vi "sub_Main Robot.vi"() -> ()   [LabVIEW 2017]
uses:
  <vilib>/Analysis/Matrix/Datatypes/RealMatrix.ctl
  <vilib>/Analysis/baseanly.llb/Mean (DBL).vi
  <vilib>/Analysis/baseanly.llb/A x Vector.vi
  <vilib>/DAQmx/read.llb/DAQmx Read (Analog 2D DBL NChan NSamp).vi
  <vilib>/DAQmx/create/channels.llb/DAQmx Create Channel (AI-Voltage-Basic).vi
  <vilib>/DAQmx/configure/timing.llb/DAQmx Timing (Sample Clock).vi
  <vilib>/DAQmx/miscellaneous.llb/DAQmx Fill In Error Info.vi
  <vilib>/Analysis/3filter.llb/Butterworth Filter (DBL).vi
  <vilib>/Analysis/NI_AALBase.lvlib
  <vilib>/Analysis/Matrix/NI_Matrix.lvlib
panel:
  in  "Calibration Matrix":T1
  out "Waveform Chart":T2(graph)
  out "Waveform Graph":dbl[][](graph)
  in  "stop":bool
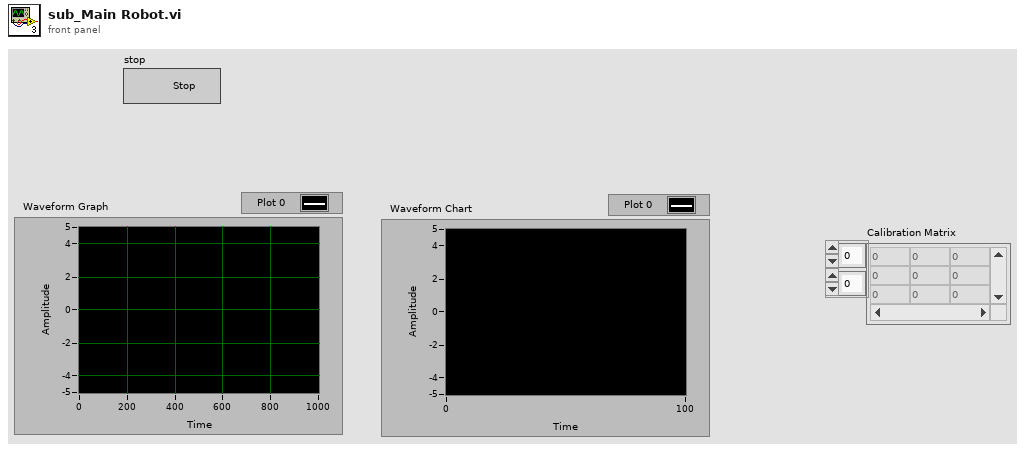
[diagram p1: front panel]
types:
  T1 = typedef "NI_Matrix.lvlib/RealMatrix.ctl" = dbl[][]
  T2 = cluster{"mean":dbl, "mean":dbl, "mean":dbl, "mean":dbl, "mean":dbl, "mean":dbl}
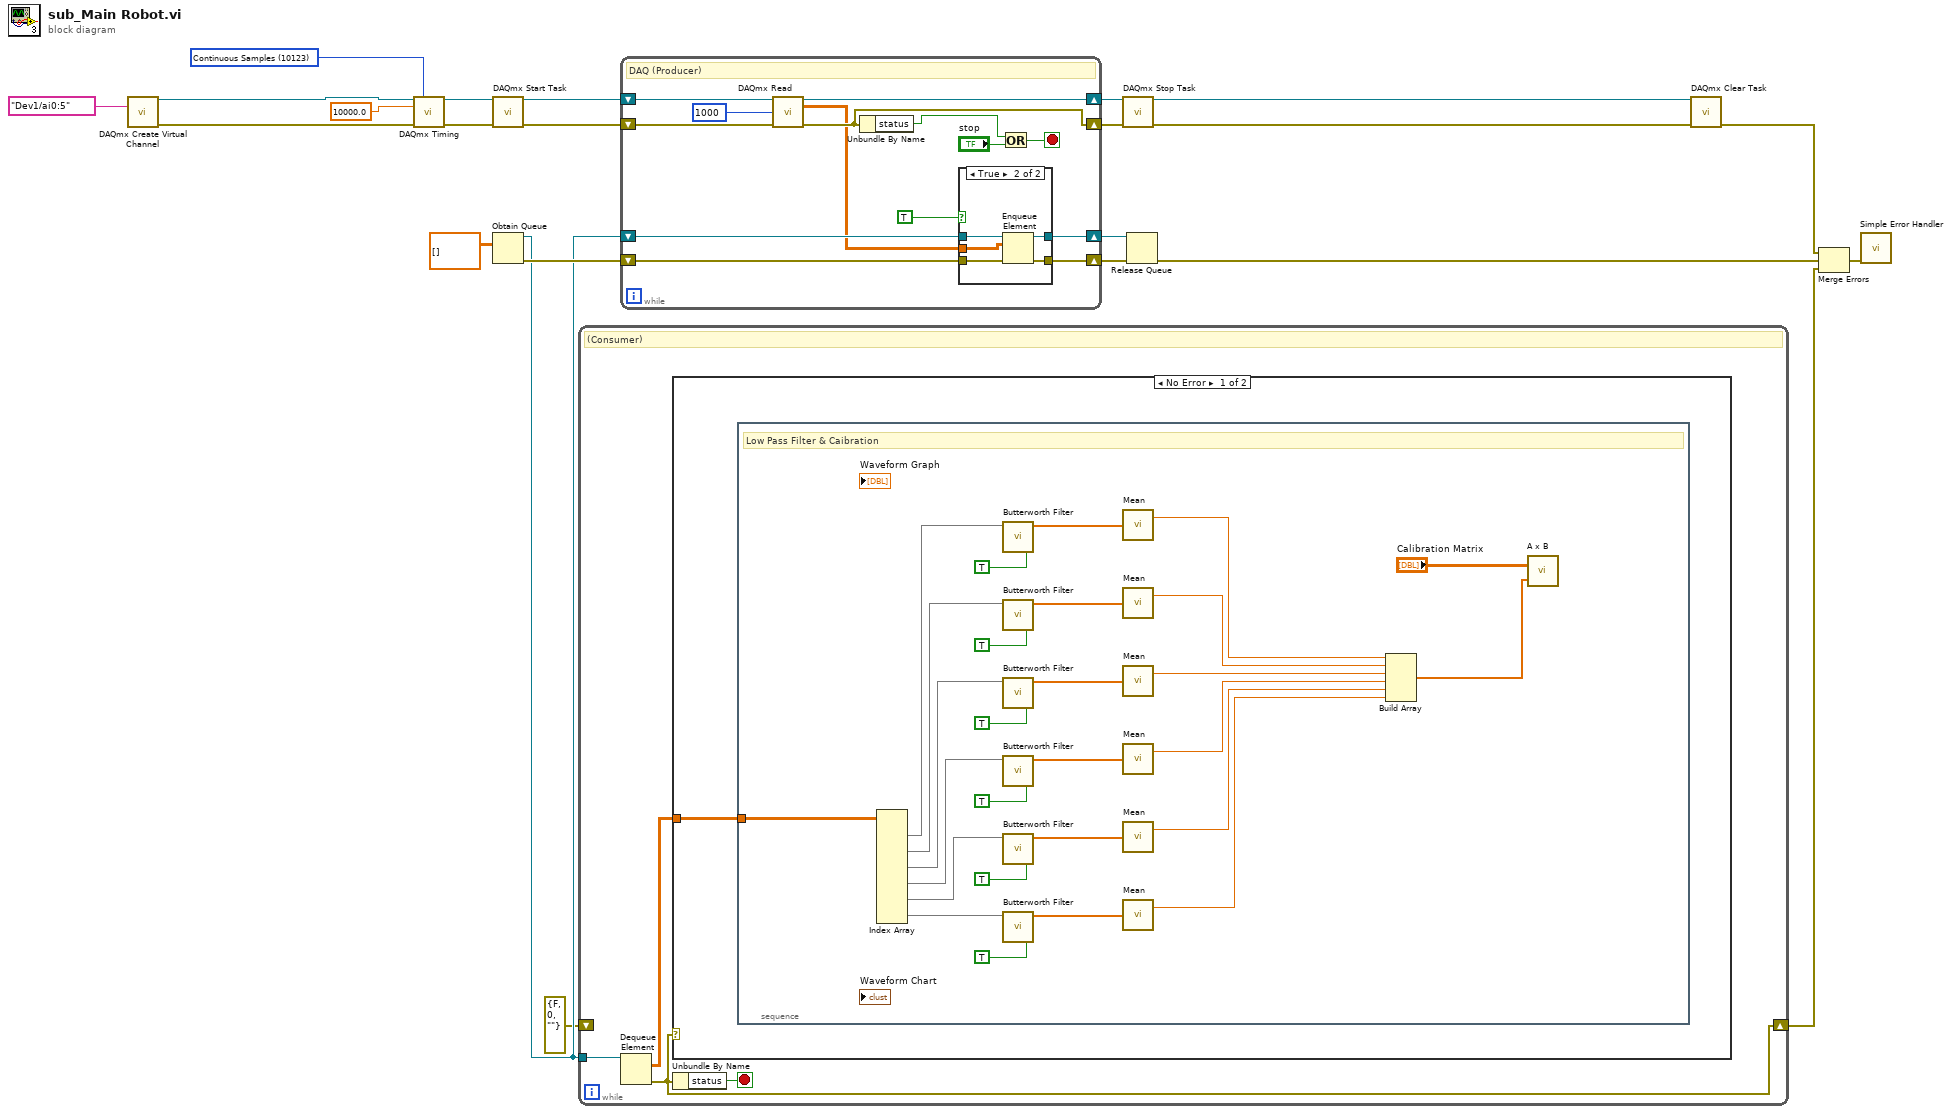
[diagram p0: block diagram]
diagram:
  w11 = 10123 items=["Finite Samples"=10178, "Continuous Samples"=10123, "Hardware Timed Single Point"=12522] ("sample mode")
  n1 = call-poly <vilib>:"DAQmx Create Virtual Channel.vi"("physical channels"=tag "Dev1/ai0:5") -> ("task out"=w22:refnum<k21>, "error out"=w21:errorcluster)  [unwired: 13 in]
  n2 = call-poly <vilib>:"DAQmx Timing.vi"("task/channels in"=w22, "sample mode"=w11, "rate"=10000.0, "error in"=w21) -> ("task out"=w19:refnum<k21>, "error out"=w20:errorcluster)  [unwired: 10 in]
  n3 = call <vilib>:"DAQmx Start Task.vi"("task/channels in"=w19, "error in"=w20) -> ("task out"=w18:refnum<k21>, "error out"=w15:errorcluster)  [unwired: 12 in]
  n4 = Obtain Queue(element data type=dbl[][] [] ("data")) -> (queue out=w6:refnum<queue>, error out=w10:errorcluster)  [unwired: 4 in, 1 out]
  n5 = while {
    tunnel: w6 -> [w27]
    shift-right: [w24] -> w1
    shift-left: errorcluster {"status"=FALSE, "code"=0, "source"=""} ("error out") -> [_]
    stop <- w26 stop-if-true
    # "(Consumer)"
    n6 = Dequeue Element(queue=w27) -> (element=w25:dbl[][], error out=w24:errorcluster)  [unwired: 2 in, 2 out]
    n7 = case shown="No Error" w24 {
      tunnel: w25 -> [w28 _]
      frame No Error {
        n8 = stacked-sequence {
          tunnel: w28 -> [w54]
          frame #0 {
            # "Low Pass Filter & Caibration"
            n9 = Index Array(array=w54) -> (element #1=w55:dbl[], element #2=w53:dbl[], element #3=w52:dbl[], element #4=w51:dbl[], element #5=w50:dbl[], element #6=w49:dbl[])  [unwired: 12 in]
            n10 = call-poly <vilib>:"Butterworth Filter.vi"("init/cont (init:F)"=TRUE, "X"=w55) -> ("Filtered X"=w48:dbl[])  [unwired: 6 in, 1 out]
            n11 = call-poly <vilib>:"Butterworth Filter.vi"("init/cont (init:F)"=TRUE, "X"=w53) -> ("Filtered X"=w47:dbl[])  [unwired: 6 in, 1 out]
            n12 = call-poly <vilib>:"Butterworth Filter.vi"("init/cont (init:F)"=TRUE, "X"=w52) -> ("Filtered X"=w46:dbl[])  [unwired: 6 in, 1 out]
            n13 = call-poly <vilib>:"Butterworth Filter.vi"("init/cont (init:F)"=TRUE, "X"=w51) -> ("Filtered X"=w45:dbl[])  [unwired: 6 in, 1 out]
            n14 = call-poly <vilib>:"Butterworth Filter.vi"("init/cont (init:F)"=TRUE, "X"=w50) -> ("Filtered X"=w44:dbl[])  [unwired: 6 in, 1 out]
            n15 = call-poly <vilib>:"Butterworth Filter.vi"("init/cont (init:F)"=TRUE, "X"=w49) -> ("Filtered X"=w43:dbl[])  [unwired: 6 in, 1 out]
            n16 = call-poly <vilib>:"Mean.vi"("X"=w48) -> ("mean"=w42:dbl)  [unwired: 1 out]
            n17 = call-poly <vilib>:"Mean.vi"("X"=w47) -> ("mean"=w41:dbl)  [unwired: 1 out]
            n18 = call-poly <vilib>:"Mean.vi"("X"=w46) -> ("mean"=w40:dbl)  [unwired: 1 out]
            n19 = call-poly <vilib>:"Mean.vi"("X"=w45) -> ("mean"=w39:dbl)  [unwired: 1 out]
            n20 = call-poly <vilib>:"Mean.vi"("X"=w44) -> ("mean"=w38:dbl)  [unwired: 1 out]
            n21 = call-poly <vilib>:"Mean.vi"("X"=w43) -> ("mean"=w37:dbl)  [unwired: 1 out]
            n22 = Build Array(w42, w41, w40, w39, w38, w37) -> (w29:dbl[])
            n23 = call-poly <vilib>:"A x B.vi"("Vector"=w29, "A"="Calibration Matrix") -> ()  [unwired: 2 out]
          }
        }
      }
      frame Error {
      }
    }
    n24 = Unbundle By Name(w24) -> ("status"=w26:bool)
  }
  n25 = while {
    shift-right: [w60] -> w5
    shift-left: w6 -> [w61]
    shift-right: [w58] -> w4
    shift-left: w10 -> [w59]
    shift-right: [w68] -> w17
    shift-left: w18 -> [w69]
    shift-right: [w65] -> w14
    shift-left: w15 -> [w67]
    stop <- w62 stop-if-true
    # "DAQ (Producer)"
    n26 = call-poly <vilib>:"DAQmx Read.vi"("task/channels in"=w69, "number of samples per channel"=1000, "error in"=w67) -> ("task out"=w68:refnum<k21>, "data"=w56:dbl[][], "error out"=w65:errorcluster)  [unwired: 10 in]
    n27 = Unbundle By Name(w65) -> ("status"=w64:bool)
    n28 = case shown="True" TRUE ("transmit") {
      tunnel: w61 -> [w71 w76]
      tunnel: [w71 w75] -> w60
      tunnel: w59 -> [w70 w74]
      tunnel: [w70 w73] -> w58
      tunnel: w56 -> [_ w72]
      frame False {
      }
      frame True {
        n29 = Enqueue Element(queue=w76, element=w72, error in (no error)=w74) -> (queue out=w75:refnum<queue>, error out=w73:errorcluster)  [unwired: 1 in, 1 out]
      }
    }
    n30 = Or(x=w64, y="stop") -> (x .or. y?=w62:bool)
  }
  n31 = call <vilib>:"DAQmx Stop Task.vi"("task/channels in"=w17, "error in"=w14) -> ("task out"=w16:refnum<k21>, "error out"=w13:errorcluster)  [unwired: 12 in]
  n32 = Release Queue(queue=w5, error in (no error)=w4) -> (error out=w3:errorcluster)  [unwired: 1 in, 2 out]
  n33 = call <vilib>:"DAQmx Clear Task.vi"("task in"=w16, "error in"=w13) -> ("error out"=w8:errorcluster)  [unwired: 13 in]
  n34 = Merge Errors(w8, w3, w1) -> (w9:errorcluster)
  n35 = call <vilib>:"Simple Error Handler.vi"("error in (no error)"=w9) -> ()  [unwired: 4 in, 5 out]
